vi "GyroDataStreamOut.vi"(11 "MockGyroData":T1={"BufferUpdateFIFO"="MockGyroBufferUpdate", "MockGyroCommandInput"="ModbusSubnetEGyroRxDataFIFO", "MockGyroDataOutput"="ModbusSubnetEGyroTxDataFIFO", "MockGyroDataRate"="MockGyroDataRateRegister", "MockGyroXValue"="MockGyroXValueRegister", "MockGyroYValue"="MockGyroYValueRegister", "MockGyroZValue"="MockGyroZValueRegister", "MockGyroStatus"="MockGyroStatusRegister", "MockGyroTemperature"="MockGyroTemperatureRegister", "CRCDataFIFO"="MockGyroCRCDataFIFO", "CRCCalculateFIFO"="MockGyroCRCCalculateFIFO", "CRCFIFO"="MockGyroCRCFIFO", "MockGyroCommandReplyFIFO"="MockGyroCommandReplyFIFO", "MockGyroReplyReadyFIFO"="MockGyroReplyReadyFIFO", "MockGyroModeFIFO"="MockGyroModeFIFO"}) -> ()   [LabVIEW 2016, in "FPGAMockGyro.lvlib"]
uses:
  FPGAMockGyro.lvlib
  DataTypes/MockGyroData.ctl
  DataTypes/MockGyroState.ctl
  DataTypes/MockGyroStateTypes.ctl
  DataTypes/MockGyroModes.ctl
  <vilib>/Platform/TimedLoop/XDataNode/timing_clust.ctl
  <vilib>/Platform/TimedLoop/XDataNode/nitl_modes.ctl
  <vilib>/Platform/TimedLoop/XDataNode/wakeup.ctl
  <vilib>/rvi/Emulation/niFpgaSctlEmulationGetInTimedLoop.vi
  <vilib>/rvi/Emulation/niFpgaEmulationReportErrorSimple.vi
  <vilib>/rvi/Emulation/niFpgaGetClockAttributes.vi
  <vilib>/rvi/Emulation/niFpgaCriticalErrorInLSC.vi
  <vilib>/rvi/DataTransferAndStorage/Container/Common/niFpgaContainerExecOnDevCompGetState.vi
  <vilib>/rvi/Emulation/niFpgaEmulationIsFPGAContextNoSignature.vi
  <vilib>/rvi/errors/niFpgaSetErrorForExecOnDevCompSimple.vi
  <vilib>/rvi/eio/common/nirviEmuReportErrorAndStop.vi
  <vilib>/rvi/DataTransferAndStorage/Container/Common/niFpgaContainerGetUniqueNameForEmu.vi
  <vilib>/rvi/FIFO/Fifo_Resource/nirvififoEmulationSetSize.vi
  <vilib>/rvi/FIFO/Fifo_Resource/nirviFifoEmulationQueueMgr.vi
  <instcachedir>/0/nirviFifoEmulationQueueMgr_E5CAEC123FF24DC58D834DCA3CDAA9B5.lvgen/nirviFifoEmulationQueueMgr_E5CAEC123FF24DC58D834DCA3CDAA9B5_000.vi
  <vilib>/rvi/FIFO/Fifo_Resource/nirvififoEmulationDetermineInputValidOut.vi
  <vilib>/rvi/FIFO/Fifo_Resource/nirvififoEmulationCreateLock.vi
  <vilib>/rvi/Emulation/niFpgaProcessEmulError.vi
  <vilib>/rvi/FIFO/Fifo_Resource/nirvififoEmulationObtainLock.vi
  <vilib>/rvi/FIFO/Fifo_Resource/nirvififoEmulationReleaseLock.vi
  <vilib>/rvi/occurrence/nirviWaitOnOccurrenceBase.vi
  <vilib>/rvi/errors/nirviReportUnexpectedCaseInternalError.vi
  <vilib>/rvi/errors/nirviReportUnexpectedCaseInternalError (U32).vi
  <vilib>/Utility/error.llb/Clear Errors.vi
  <vilib>/rvi/interface/RandomDataEmulation/niFpgaRandomDataHandleErrors.vi
  <vilib>/rvi/Memory/Memory_Emulation/niFpgaMemoryEmulationCacheClearOnFirstRun.vi
  <vilib>/rvi/Memory/Memory_Emulation/nirvimemoryEmulationManagerCache_MakeExclusive.vi
  <vilib>/rvi/Memory/Memory_Emulation/niFpgaMemoryEmulationValidateCache.vi
  <vilib>/rvi/Memory/Memory_Emulation/nirvimemoryEmulationManagerCache_InsertValue.vi
  <vilib>/rvi/Memory/Memory_Emulation/nirvimemoryEmulationManagerCache_ReleaseExclusive.vi
  <vilib>/rvi/Memory/Memory_Emulation/nirvimemoryEmulationManagerCache_GetValue.vi
  <vilib>/rvi/Memory/Memory_Emulation/nirvimemoryEmulationManagerCache_SetValue.vi
  <instcachedir>/0/nirviFifoEmulationQueueMgr_E5CAEC123FF24DC58D834DCA3CDAA9B5.lvgen/nirviFifoEmulationQueueMgr_E5CAEC123FF24DC58D834DCA3CDAA9B5_002.vi
  <instcachedir>/0/nirviFifoEmulationQueueMgr_E5CAEC123FF24DC58D834DCA3CDAA9B5.lvgen/nirviFifoEmulationQueueMgr_E5CAEC123FF24DC58D834DCA3CDAA9B5_001.vi
  <vilib>/Platform/TimedLoop/XDataNode/XDataNode.xnode
  <vilib>/rvi/DataTransferAndStorage/Container/XNode/niFpgaContainer.xnode
  <vilib>/rvi/FIFO/Fifo_Resource/niFpgaFifoEmulationRefIn.vi
  <vilib>/rvi/DataTransferAndStorage/Register/Emulation/niFpgaRegisterEmulationRefIn.vi
  <vilib>/Platform/TimedLoop/XDataNode/XDNodeRunTimeDep.lvlib
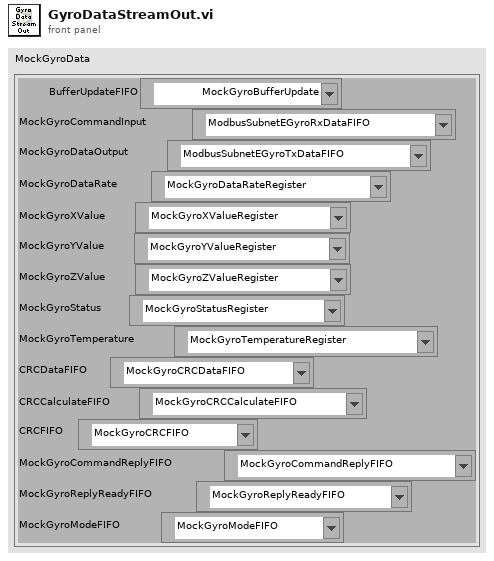
[diagram p1: front panel]
types:
  T1 = typedef "FPGAMockGyro.lvlib/MockGyroData.ctl" = cluster{"BufferUpdateFIFO":refnum<k21>, "MockGyroCommandInput":refnum<k21>, "MockGyroDataOutput":refnum<k21>, "MockGyroDataRate":refnum<k21>, "MockGyroXValue":refnum<k21>, "MockGyroYValue":refnum<k21>, "MockGyroZValue":refnum<k21>, "MockGyroStatus":refnum<k21>, "MockGyroTemperature":refnum<k21>, "CRCDataFIFO":refnum<k21>, "CRCCalculateFIFO":refnum<k21>, "CRCFIFO":refnum<k21>, "MockGyroCommandReplyFIFO":refnum<k21>, "MockGyroReplyReadyFIFO":refnum<k21>, "MockGyroModeFIFO":refnum<k21>}
  T2 = typedef "FPGAMockGyro.lvlib/MockGyroState.ctl" = cluster{"MockGyroStateTypes":T3, "DelayTicks":u64, "NextDelayTicks":u64, "Index":i32, "DataOutputArray":u8[], "MockGyroModes":T4}
  T3 = typedef "FPGAMockGyro.lvlib/MockGyroStateTypes.ctl" = enum8{"Processing", "WriteXValues", "WriteYValues", "WriteZValues", "WriteTemperature", "WriteDataOutput", "WriteCRC32", "Delaying", "CheckCommandReply", "WriteCommandReply", "Config"}
  T4 = typedef "FPGAMockGyro.lvlib/MockGyroModes.ctl" = enum8{"Normal", "Config"}
  T5 = typedef "XDNodeRunTimeDep.lvlib/timing_clust.ctl" = cluster{"Expected End [f-1]":u64, "Actual End [f-1]":u64, "Finished Late? [f-1]":bool, "Expected End [i-1]":u64, "Actual End [i-1]":u64, "Finished Late? [i-1]":bool, "Expected Start [i]":u64, "Actual Start [i]":u64, "Expected Start [f]":u64, "Actual Start [f]":u64, "Source Name":string, "Structure Name":string, "Period":i64, "Deadline":i64, "Offset":i64, "Start":i64, "Priority":i32, "Timeout":i32, "Mode":T6, "Wakeup Reason":T7, "Error":errorcluster, "Source Type":string, "Secondary Source Type":string, "Global End Time":u64, "Global Start Time":u64, "Frame Duration":u64, "Iteration Duration":u64, "Assigned CPU":i32, "I/O Scan Engine Mode":u32}
  T6 = typedef "XDNodeRunTimeDep.lvlib/nitl_modes.ctl" = enum32{"No Change", "Process missed periods, maintain original phase", "Discard missed periods, maintain original phase", "Process missed periods, ignore original phase", "Discard missed periods, ignore original phase"}
  T7 = typedef "XDNodeRunTimeDep.lvlib/wakeup.ctl" = enum32{"Normal", "Aborted", "Asynchronous wakeup", "Timing source error", "Timed loop error", "Timeout"}
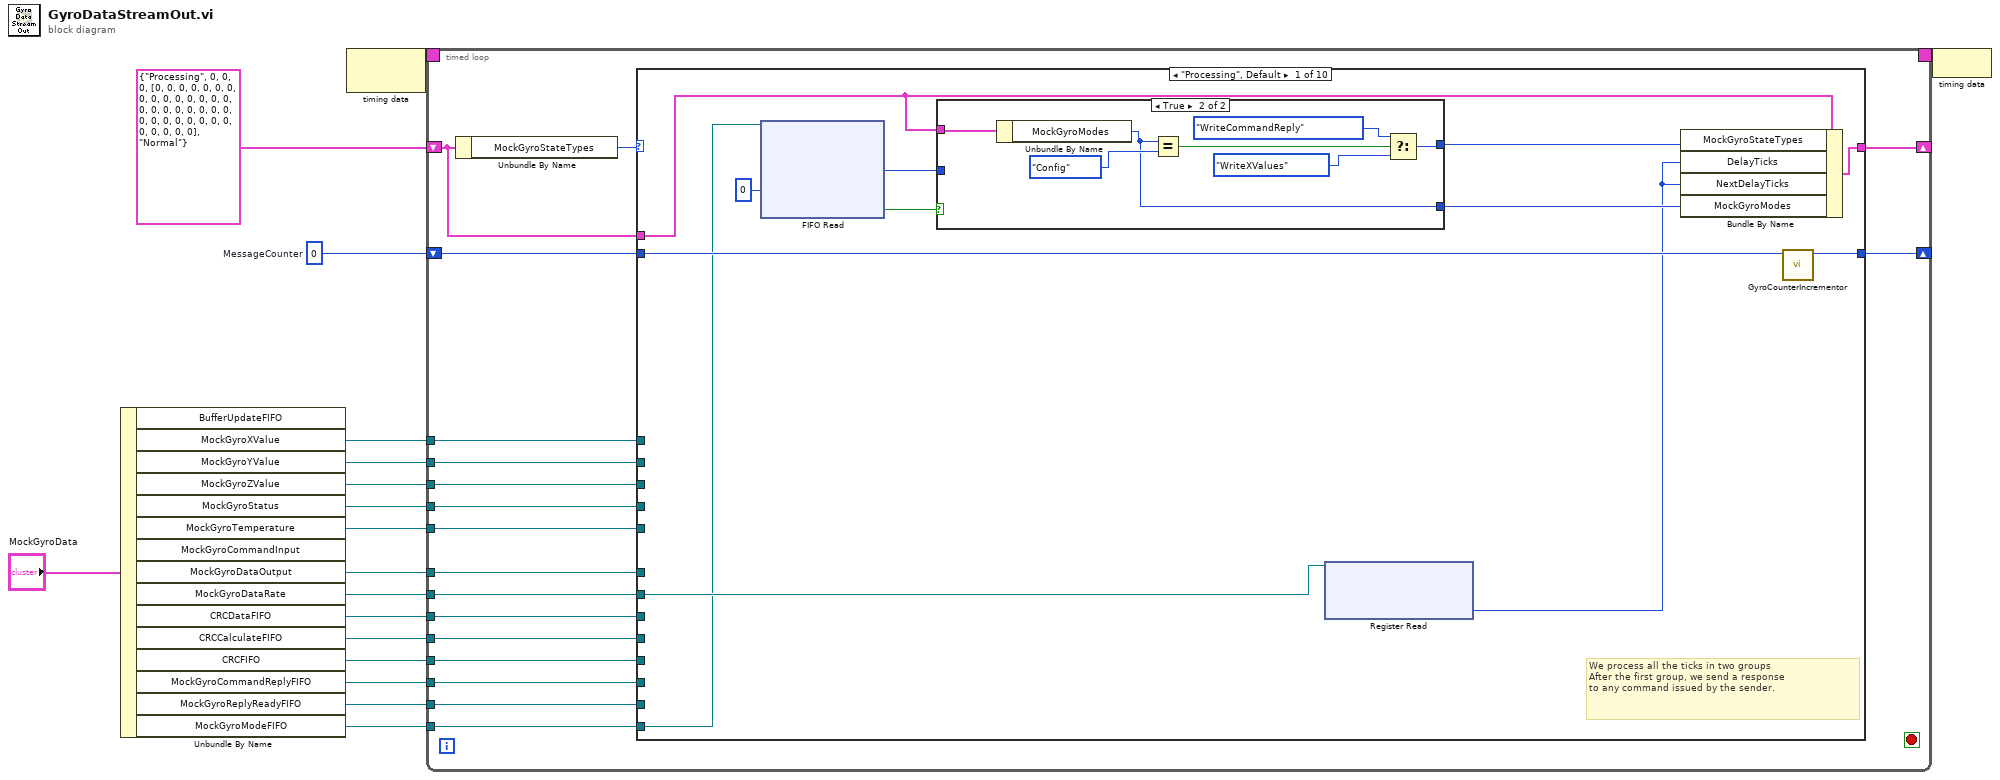
[diagram p0: block diagram]
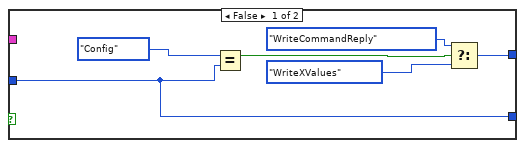
[diagram p2: hidden frame]
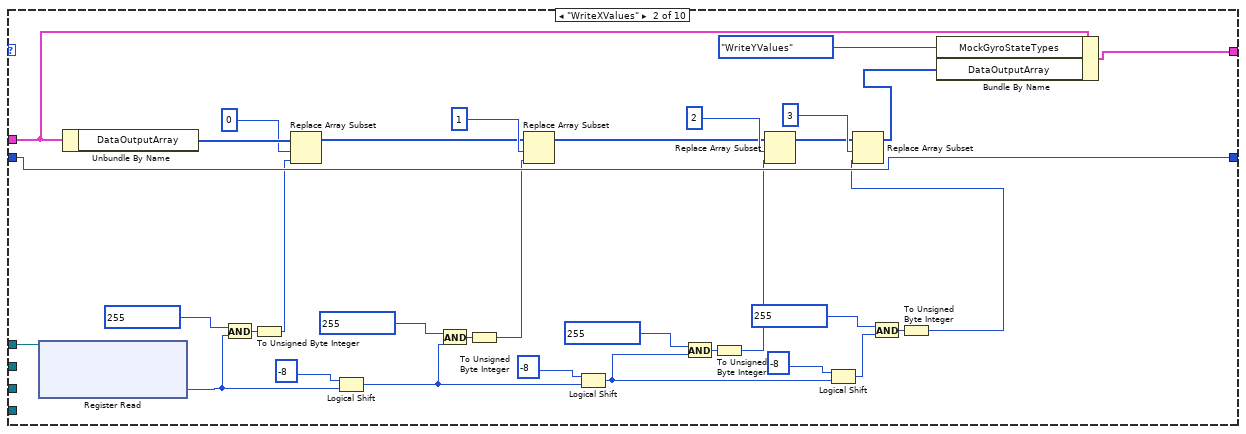
[diagram p3: hidden frame]
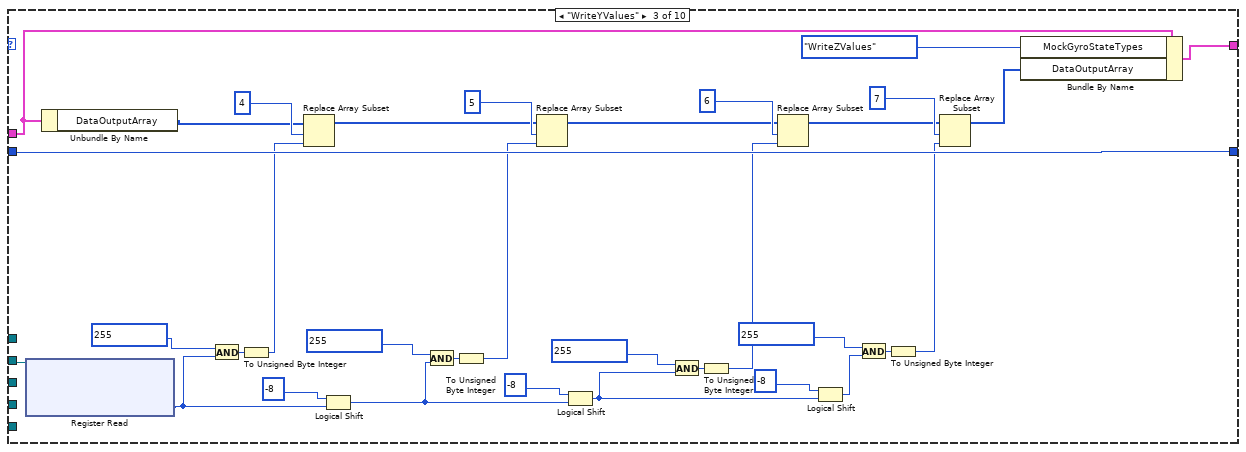
[diagram p4: hidden frame]
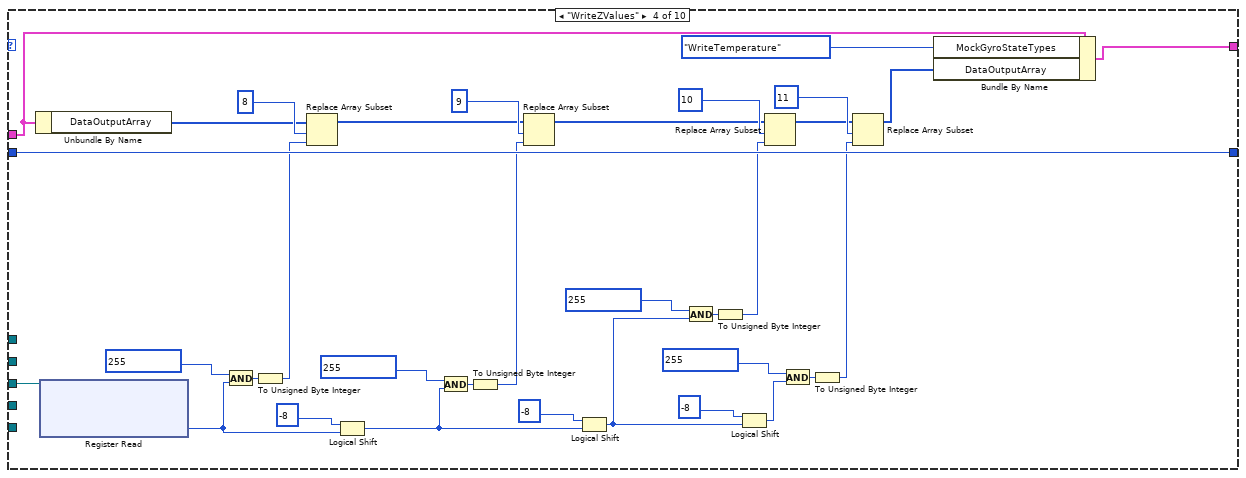
[diagram p5: hidden frame]
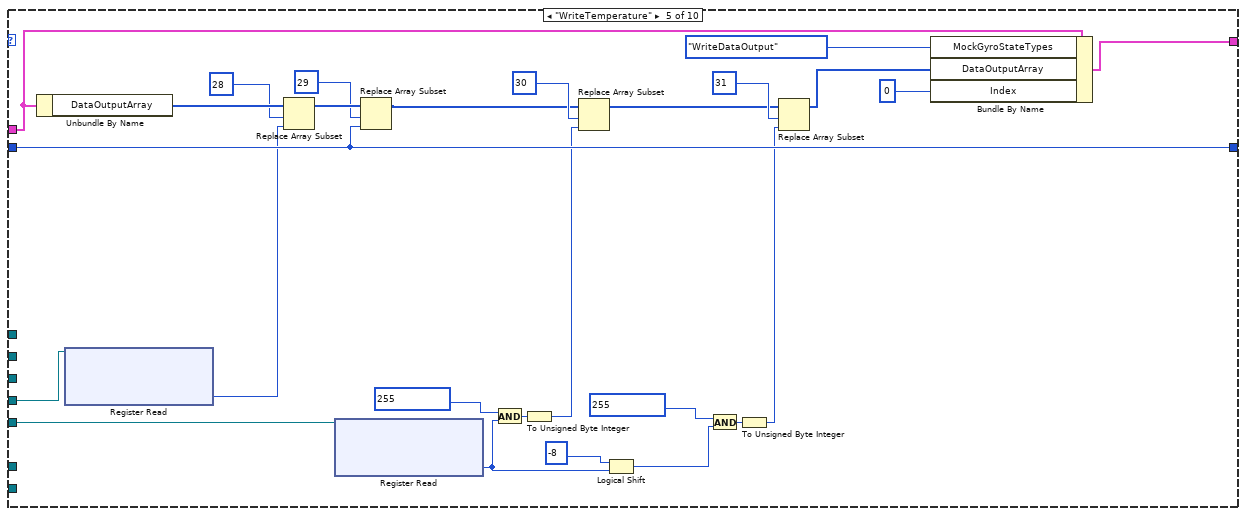
[diagram p6: hidden frame]
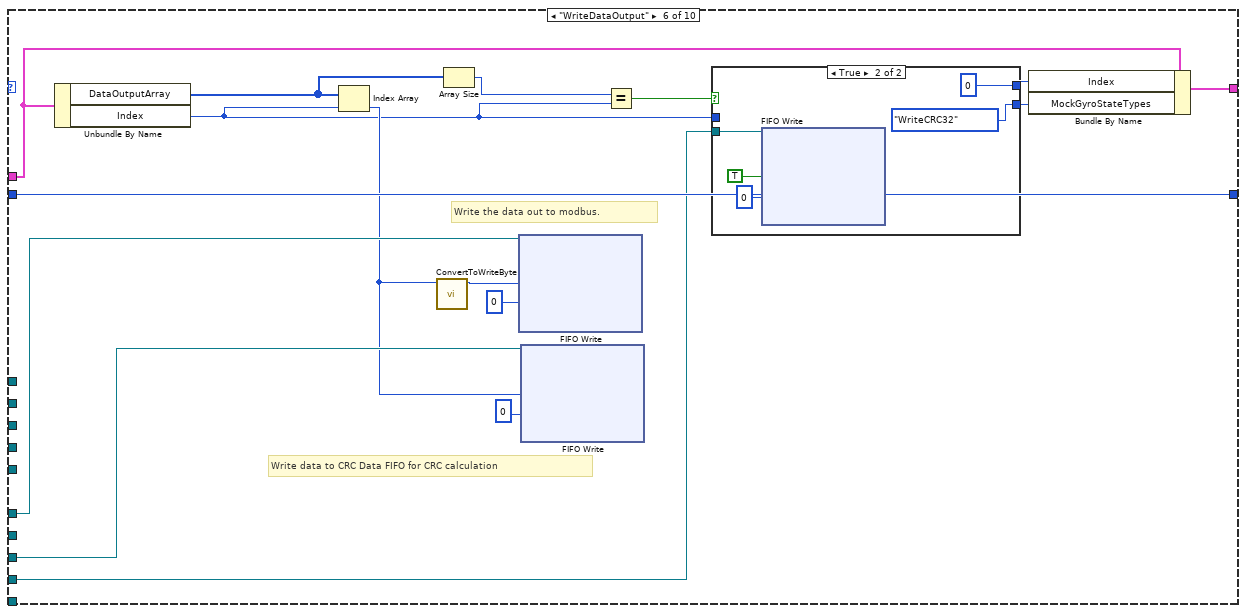
[diagram p7: hidden frame]
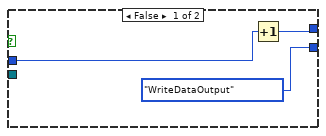
[diagram p8: hidden frame]
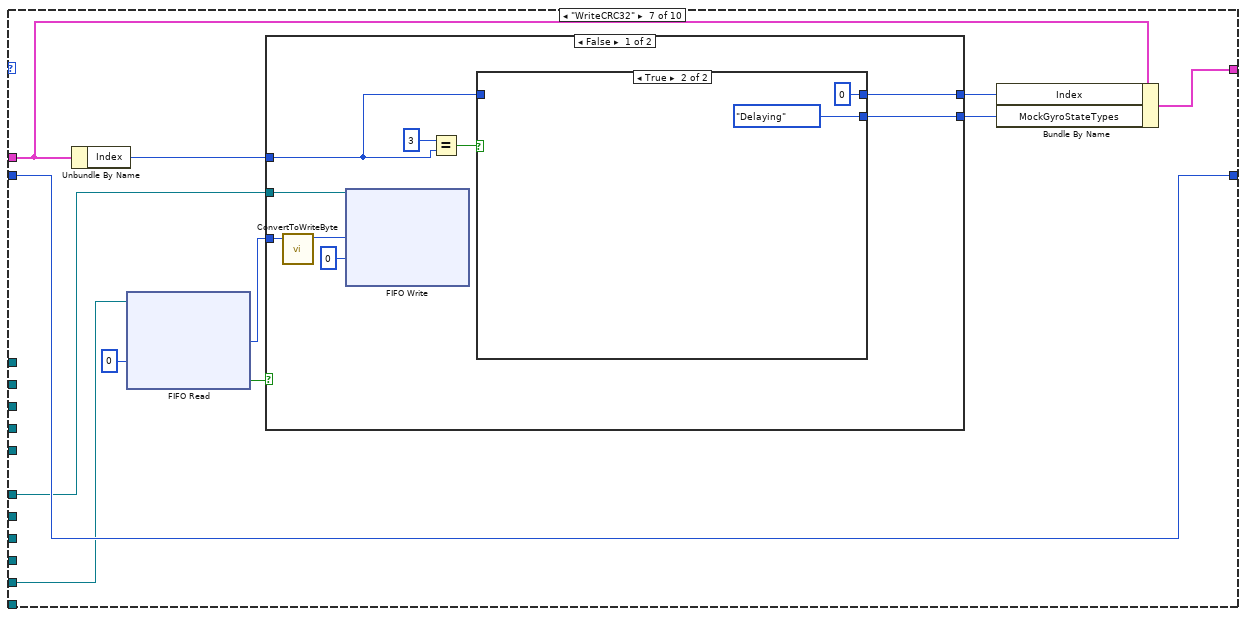
[diagram p9: hidden frame]
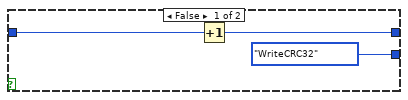
[diagram p10: hidden frame]
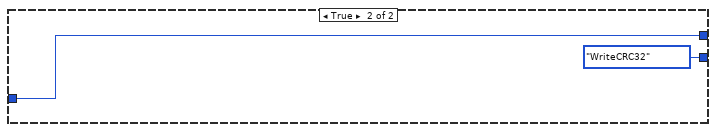
[diagram p11: hidden frame]
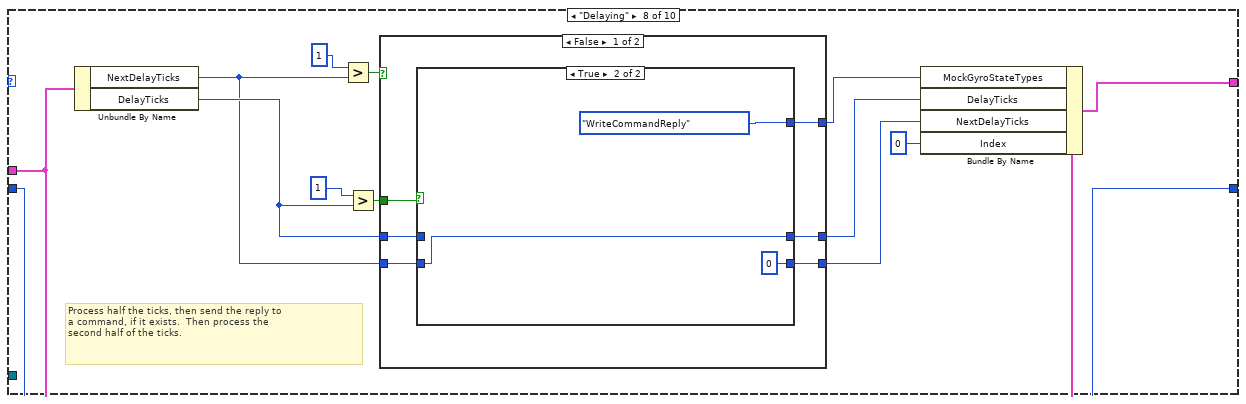
[diagram p12: hidden frame]
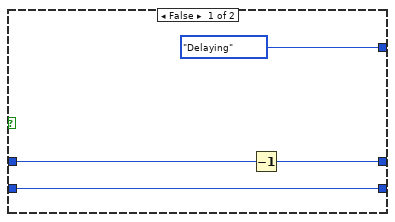
[diagram p13: hidden frame]
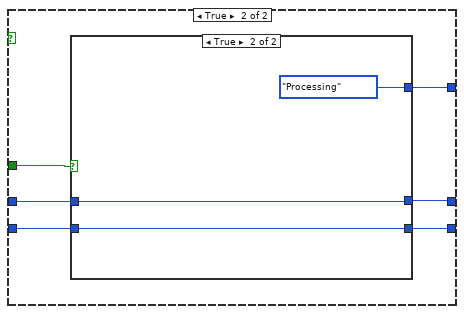
[diagram p14: hidden frame]
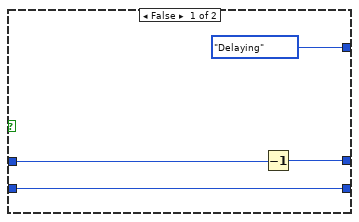
[diagram p15: hidden frame]
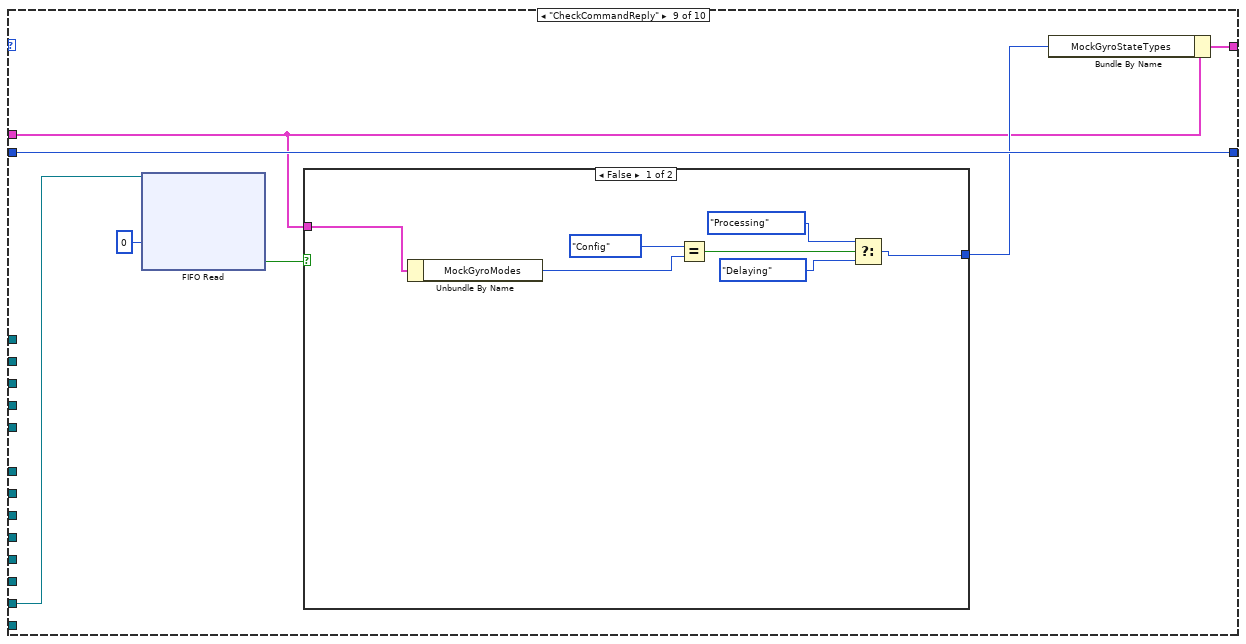
[diagram p16: hidden frame]
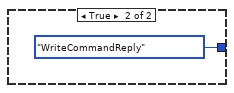
[diagram p17: hidden frame]
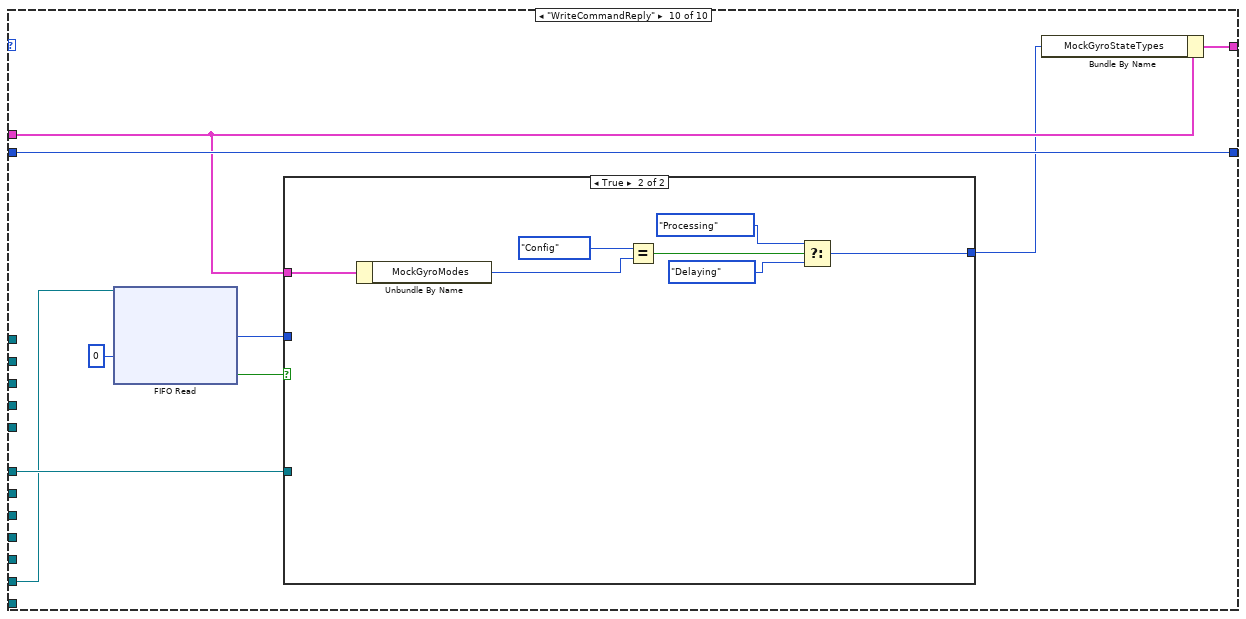
[diagram p18: hidden frame]
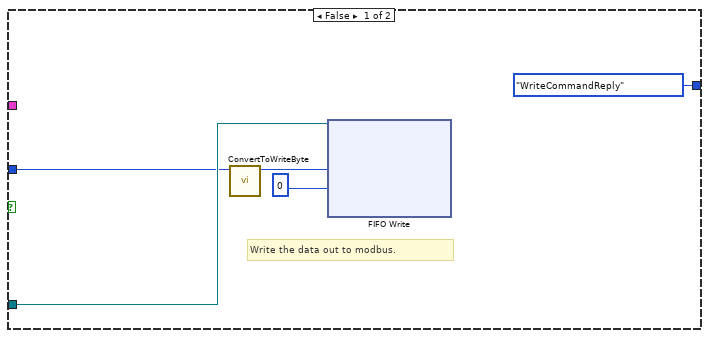
[diagram p19: hidden frame]
diagram:
  w18 = u8 0  # MessageCounter
  n1 = Unbundle By Name("MockGyroData") -> ("MockGyroXValue"=w11:refnum<k21>, "MockGyroYValue"=w10:refnum<k21>, "MockGyroZValue"=w9:refnum<k21>, "MockGyroStatus"=w8:refnum<k21>, "MockGyroTemperature"=w7:refnum<k21>, "MockGyroDataOutput"=w13:refnum<k21>, "MockGyroDataRate"=w14:refnum<k21>, "CRCDataFIFO"=w6:refnum<k21>, "CRCCalculateFIFO"=w5:refnum<k21>, "CRCFIFO"=w4:refnum<k21>, "MockGyroCommandReplyFIFO"=w3:refnum<k21>, "MockGyroReplyReadyFIFO"=w2:refnum<k21>, "MockGyroModeFIFO"=w1:refnum<k21>)  [unwired: 2 out]
  n2 = node-c288() -> (w16:T5)  [unwired: 1 in]
  n3 = timed-loop {
    shift-right: [w32] -> _
    shift-left: T2 {"MockGyroStateTypes"=enum."Processing", "DelayTicks"=0, "NextDelayTicks"=0, "Index"=0, "DataOutputArray"=[0, 0, 0, 0, 0, 0, 0, 0, 0, 0, 0, 0, 0, 0, 0, 0, 0, 0, 0, 0, 0, 0, 0, 0, 0, 0, 0, 0, 0, 0, 0, 0, 0, 0, 0, 0], "MockGyroModes"=enum."Normal"} ("MockGyroState") -> [w33]
    shift-right: [w36] -> _
    shift-left: w18 -> [w35]
    timing: w16 -> [_]
    timing-out: [_] -> w15
    tunnel: w14 -> [w31]
    tunnel: w13 -> [w30]
    tunnel: w11 -> [w29]
    tunnel: w10 -> [w28]
    tunnel: w9 -> [w27]
    tunnel: w8 -> [w26]
    tunnel: w7 -> [w25]
    tunnel: w6 -> [w24]
    tunnel: w5 -> [w23]
    tunnel: w4 -> [w22]
    tunnel: w3 -> [w21]
    tunnel: w2 -> [w20]
    tunnel: w1 -> [w19]
    stop <- _ stop-if-true
    n4 = Unbundle By Name(w33) -> ("MockGyroStateTypes"=w34:T3)
    n5 = case shown="\"Processing\", Default" w34 {
      tunnel: [w48 w83 w120 w153 w181 w196 w220 w250 w280 w298] -> w36
      tunnel: w35 -> [w47 w83 w120 w153 w181 w196 w220 w250 w280 w298]
      tunnel: w33 -> [w39 w86 w118 w151 w186 w195 w221 w249 w277 w293]
      tunnel: [w46 w85 w116 w149 w185 w197 w211 w248 w279 w299] -> w32
      tunnel: w31 -> [w44 _ _ _ _ _ _ _ _ _]
      tunnel: w30 -> [_ _ _ _ _ w200 w213 _ _ w300]
      tunnel: w29 -> [_ w81 _ _ _ _ _ _ _ _]
      tunnel: w28 -> [_ _ w99 _ _ _ _ _ _ _]
      tunnel: w27 -> [_ _ _ w132 _ _ _ _ _ _]
      tunnel: w26 -> [_ _ _ _ w163 _ _ _ _ _]
      tunnel: w25 -> [_ _ _ _ w166 _ _ _ _ _]
      tunnel: w24 -> [_ _ _ _ _ w194 _ _ _ _]
      tunnel: w23 -> [_ _ _ _ _ w187 _ _ _ _]
      tunnel: w22 -> [_ _ _ _ _ _ w216 _ _ _]
      tunnel: w21 -> [_ _ _ _ _ _ _ _ _ w297]
      tunnel: w20 -> [_ _ _ _ _ _ _ _ w283 _]
      tunnel: w19 -> [w43 _ _ _ _ _ _ _ _ _]
      frame "Processing", Default {
        # "We process all the ticks in two groups\nAfter the first group, we send a response\nto any command issued by the sender."
        n6 = xnode ("FIFO Read")("Timeout"=0, "FIFO In"=w43) -> ("Element"=w40:u8, "Timed Out?"=w41:bool)  [unwired: 1 out]
        n7 = case shown="True" w41 {
          tunnel: [w51 w55] -> w45
          tunnel: w40 -> [w49 _]
          tunnel: w39 -> [_ w60]
          tunnel: [w49 w56] -> w38
          frame False {
            n8 = Equal?(x=MockGyroModes."Config" ("MockGyroModes"), y=w49) -> (x = y?=w54:bool)
            n9 = Select(t=MockGyroStateTypes."WriteCommandReply" ("MockGyroStateTypes"), s=w54, f=MockGyroStateTypes."WriteXValues") -> (s? t:f=w51:T3)
          }
          frame True {
            n10 = Unbundle By Name(w60) -> ("MockGyroModes"=w56:T4)
            n11 = Equal?(x=w56, y=MockGyroModes."Config" ("MockGyroModes")) -> (x = y?=w61:bool)
            n12 = Select(t=MockGyroStateTypes."WriteCommandReply" ("f"), s=w61, f=MockGyroStateTypes."WriteXValues") -> (s? t:f=w55:T3)
          }
        }
        n13 = xnode ("Register Read")("Register In"=w44) -> ("Data"=w37:u64)  [unwired: 1 out]
        n14 = Bundle By Name(cluster=w39, "MockGyroStateTypes"=w45, "DelayTicks"=w37, "NextDelayTicks"=w37, "MockGyroModes"=w38) -> (w46:T2)
        n15 = call "GyroCounterIncrementor.vi"("CurrentCounter"=w47) -> ("NewCounter"=w48:u8)  [unwired: 10 in]
      }
      frame "WriteXValues" {
        n16 = xnode ("Register Read")("Register In"=w81) -> ("Data"=w78:u32)  [unwired: 1 out]
        n17 = Unbundle By Name(w86) -> ("DataOutputArray"=w94:u8[])
        n18 = And(x=u32 255, y=w78) -> (x .and. y?=w79:u32)
        n19 = To Unsigned Byte Integer(number=w79) -> (unsigned 8bit integer=w76:u8)
        n20 = Replace Array Subset(array=w94, new element=w76, index=0) -> (w89:u8[])
        n21 = Logical Shift(y=i16 -8, x=w78) -> (x << y=w71:u32)
        n22 = And(x=u32 255, y=w71) -> (x .and. y?=w74:u32)
        n23 = To Unsigned Byte Integer(number=w74) -> (unsigned 8bit integer=w73:u8)
        n24 = Replace Array Subset(array=w89, new element=w73, index=1) -> (w88:u8[])
        n25 = Logical Shift(y=i16 -8, x=w71) -> (x << y=w64:u32)
        n26 = And(x=u32 255, y=w64) -> (x .and. y?=w70:u32)
        n27 = To Unsigned Byte Integer(number=w70) -> (unsigned 8bit integer=w65:u8)
        n28 = Replace Array Subset(array=w88, new element=w65, index=2) -> (w87:u8[])
        n29 = Logical Shift(y=i16 -8, x=w64) -> (x << y=w63:u32)
        n30 = And(x=u32 255, y=w63) -> (x .and. y?=w67:u32)
        n31 = To Unsigned Byte Integer(number=w67) -> (unsigned 8bit integer=w62:u8)
        n32 = Replace Array Subset(array=w87, new element=w62, index=3) -> (w84:u8[])
        n33 = Bundle By Name(cluster=w86, "MockGyroStateTypes"=MockGyroStateTypes."WriteYValues", "DataOutputArray"=w84) -> (w85:T2)
      }
      frame "WriteYValues" {
        n34 = xnode ("Register Read")("Register In"=w99) -> ("Data"=w112:u32)  [unwired: 1 out]
        n35 = Unbundle By Name(w118) -> ("DataOutputArray"=w119:u8[])
        n36 = And(x=u32 255, y=w112) -> (x .and. y?=w113:u32)
        n37 = To Unsigned Byte Integer(number=w113) -> (unsigned 8bit integer=w98:u8)
        n38 = Replace Array Subset(array=w119, new element=w98, index=4) -> (w123:u8[])
        n39 = Logical Shift(y=i16 -8, x=w112) -> (x << y=w107:u32)
        n40 = And(x=u32 255, y=w107) -> (x .and. y?=w109:u32)
        n41 = To Unsigned Byte Integer(number=w109) -> (unsigned 8bit integer=w97:u8)
        n42 = Replace Array Subset(array=w123, new element=w97, index=5) -> (w122:u8[])
        n43 = Logical Shift(y=i16 -8, x=w107) -> (x << y=w101:u32)
        n44 = And(x=u32 255, y=w101) -> (x .and. y?=w106:u32)
        n45 = To Unsigned Byte Integer(number=w106) -> (unsigned 8bit integer=w96:u8)
        n46 = Replace Array Subset(array=w122, new element=w96, index=6) -> (w121:u8[])
        n47 = Logical Shift(y=i16 -8, x=w101) -> (x << y=w100:u32)
        n48 = And(x=u32 255, y=w100) -> (x .and. y?=w103:u32)
        n49 = To Unsigned Byte Integer(number=w103) -> (unsigned 8bit integer=w95:u8)
        n50 = Replace Array Subset(array=w121, new element=w95, index=7) -> (w117:u8[])
        n51 = Bundle By Name(cluster=w118, "MockGyroStateTypes"=MockGyroStateTypes."WriteZValues", "DataOutputArray"=w117) -> (w116:T2)
      }
      frame "WriteZValues" {
        n52 = Unbundle By Name(w151) -> ("DataOutputArray"=w152:u8[])
        n53 = xnode ("Register Read")("Register In"=w132) -> ("Data"=w145:u32)  [unwired: 1 out]
        n54 = And(x=u32 255, y=w145) -> (x .and. y?=w146:u32)
        n55 = To Unsigned Byte Integer(number=w146) -> (unsigned 8bit integer=w131:u8)
        n56 = Replace Array Subset(array=w152, new element=w131, index=8) -> (w156:u8[])
        n57 = Logical Shift(y=i16 -8, x=w145) -> (x << y=w140:u32)
        n58 = And(x=u32 255, y=w140) -> (x .and. y?=w142:u32)
        n59 = To Unsigned Byte Integer(number=w142) -> (unsigned 8bit integer=w130:u8)
        n60 = Replace Array Subset(array=w156, new element=w130, index=9) -> (w155:u8[])
        n61 = Logical Shift(y=i16 -8, x=w140) -> (x << y=w134:u32)
        n62 = And(x=u32 255, y=w134) -> (x .and. y?=w139:u32)
        n63 = To Unsigned Byte Integer(number=w139) -> (unsigned 8bit integer=w129:u8)
        n64 = Logical Shift(y=i16 -8, x=w134) -> (x << y=w133:u32)
        n65 = Replace Array Subset(array=w155, new element=w129, index=10) -> (w154:u8[])
        n66 = And(x=u32 255, y=w133) -> (x .and. y?=w136:u32)
        n67 = To Unsigned Byte Integer(number=w136) -> (unsigned 8bit integer=w128:u8)
        n68 = Replace Array Subset(array=w154, new element=w128, index=11) -> (w150:u8[])
        n69 = Bundle By Name(cluster=w151, "MockGyroStateTypes"=MockGyroStateTypes."WriteTemperature", "DataOutputArray"=w150) -> (w149:T2)
      }
      frame "WriteTemperature" {
        n70 = Unbundle By Name(w186) -> ("DataOutputArray"=w183:u8[])
        n71 = xnode ("Register Read")("Register In"=w163) -> ("Data"=w162:u8)  [unwired: 1 out]
        n72 = Replace Array Subset(array=w183, new element=w162, index=28) -> (w180:u8[])
        n73 = xnode ("Register Read")("Register In"=w166) -> ("Data"=w171:u16)  [unwired: 1 out]
        n74 = Replace Array Subset(array=w180, new element=w181, index=29) -> (w176:u8[])
        n75 = And(x=u16 255, y=w171) -> (x .and. y?=w172:u16)
        n76 = To Unsigned Byte Integer(number=w172) -> (unsigned 8bit integer=w164:u8)
        n77 = Replace Array Subset(array=w176, new element=w164, index=30) -> (w175:u8[])
        n78 = Logical Shift(y=i16 -8, x=w171) -> (x << y=w167:u16)
        n79 = And(x=u16 255, y=w167) -> (x .and. y?=w168:u16)
        n80 = To Unsigned Byte Integer(number=w168) -> (unsigned 8bit integer=w165:u8)
        n81 = Replace Array Subset(array=w175, new element=w165, index=31) -> (w174:u8[])
        n82 = Bundle By Name(cluster=w186, "MockGyroStateTypes"=MockGyroStateTypes."WriteDataOutput", "DataOutputArray"=w174, "Index"=u8 0) -> (w185:T2)
      }
      frame "WriteDataOutput" {
        # "Write data to CRC Data FIFO for CRC calculation"
        # "Write the data out to modbus."
        n83 = Unbundle By Name(w195) -> ("DataOutputArray"=w198:u8[], "Index"=w188:i32)
        n84 = Index Array(array=w198, index=w188) -> (element=w192:u8)
        n85 = call "ConvertToWriteByte.vi"("Input"=w192) -> ("Output"=w199:u16)  [unwired: 10 in]
        n86 = Array Size(array=w198) -> (size(s)=w202:i32)
        n87 = xnode ("FIFO Write")("Element"=w199, "Timeout"=0, "FIFO In"=w200) -> ()  [unwired: 2 out]
        n88 = xnode ("FIFO Write")("Element"=w192, "Timeout"=0, "FIFO In"=w194) -> ()  [unwired: 2 out]
        n89 = Equal?(x=w202, y=w188) -> (x = y?=w189:bool)
        n90 = case shown="True" w189 {
          tunnel: [w203 0] -> w191
          tunnel: [MockGyroStateTypes."WriteDataOutput" ("MockGyroStateTypes") MockGyroStateTypes."WriteCRC32" ("MockGyroStateTypes")] -> w190
          tunnel: w188 -> [w204 _]
          tunnel: w187 -> [_ w208]
          frame False {
            n91 = Increment(x=w204) -> (x+1=w203:i32)
          }
          frame True {
            n92 = xnode ("FIFO Write")("Element"=TRUE, "Timeout"=0, "FIFO In"=w208) -> ()  [unwired: 2 out]
          }
        }
        n93 = Bundle By Name(cluster=w195, "Index"=w191, "MockGyroStateTypes"=w190) -> (w197:T2)
      }
      frame "WriteCRC32" {
        n94 = Unbundle By Name(w221) -> ("Index"=w219:i32)
        n95 = xnode ("FIFO Read")("Timeout"=0, "FIFO In"=w216) -> ("Element"=w212:u8, "Timed Out?"=w214:bool)  [unwired: 1 out]
        n96 = case shown="False" w214 {
          tunnel: w219 -> [w228 w237]
          tunnel: [w227 w237] -> w218
          tunnel: [w226 MockGyroStateTypes."WriteCRC32" ("MockGyroStateTypes")] -> w217
          tunnel: w213 -> [w225 _]
          tunnel: w212 -> [w223 _]
          frame False {
            n97 = call "ConvertToWriteByte.vi"("Input"=w223) -> ("Output"=w222:u16)  [unwired: 10 in]
            n98 = xnode ("FIFO Write")("Element"=w222, "Timeout"=0, "FIFO In"=w225) -> ()  [unwired: 2 out]
            n99 = Equal?(x=3, y=w228) -> (x = y?=w230:bool)
            n100 = case shown="True" w230 {
              tunnel: w228 -> [w233 _]
              tunnel: [w232 0] -> w227
              tunnel: [MockGyroStateTypes."WriteCRC32" ("MockGyroStateTypes") MockGyroStateTypes."Delaying" ("MockGyroStateTypes")] -> w226
              frame False {
                n101 = Increment(x=w233) -> (x+1=w232:i32)
              }
              frame True {
              }
            }
          }
          frame True {
          }
        }
        n102 = Bundle By Name(cluster=w221, "Index"=w218, "MockGyroStateTypes"=w217) -> (w211:T2)
      }
      frame "Delaying" {
        # "Process half the ticks, then send the reply to \na command, if it exists.  Then process the \nsecond half of the ticks."
        n103 = Unbundle By Name(w249) -> ("NextDelayTicks"=w243:u64, "DelayTicks"=w245:u64)
        n104 = Greater?(x=u64 1, y=w243) -> (0:w240:bool)
        n105 = Greater?(x=u64 1, y=w245) -> (0:w239:bool)
        n106 = case shown="False" w240 {
          tunnel: w245 -> [w256 w266]
          tunnel: [w255 w265] -> w244
          tunnel: w243 -> [w254 w267]
          tunnel: [w253 w268] -> w242
          tunnel: w239 -> [w252 w269]
          tunnel: [w251 w264] -> w238
          frame False {
            n107 = case shown="True" w252 {
              tunnel: w256 -> [w260 _]
              tunnel: [w259 w262] -> w255
              tunnel: w254 -> [w258 w262]
              tunnel: [w258 u64 0 ("NextDelayTicks")] -> w253
              tunnel: [MockGyroStateTypes."Delaying" ("f") MockGyroStateTypes."WriteCommandReply" ("MockGyroStateTypes")] -> w251
              frame False {
                n108 = Decrement(x=w260) -> (x-1=w259:u64)
              }
              frame True {
              }
            }
          }
          frame True {
            n109 = case shown="True" w269 {
              tunnel: [w273 w276] -> w268
              tunnel: w267 -> [w273 w276]
              tunnel: w266 -> [w272 w274]
              tunnel: [w271 w274] -> w265
              tunnel: [MockGyroStateTypes."Delaying" ("f") MockGyroStateTypes."Processing" ("f")] -> w264
              frame False {
                n110 = Decrement(x=w272) -> (x-1=w271:u64)
              }
              frame True {
              }
            }
          }
        }
        n111 = Bundle By Name(cluster=w249, "MockGyroStateTypes"=w238, "DelayTicks"=w244, "NextDelayTicks"=w242, "Index"=0) -> (w248:T2)
      }
      frame "CheckCommandReply" {
        n112 = xnode ("FIFO Read")("Timeout"=0, "FIFO In"=w283) -> ("Timed Out?"=w281:bool)  [unwired: 2 out]
        n113 = case shown="False" w281 {
          tunnel: [w284 MockGyroStateTypes."WriteCommandReply" ("MockGyroStateTypes")] -> w278
          tunnel: w277 -> [w285 _]
          frame False {
            n114 = Unbundle By Name(w285) -> ("MockGyroModes"=w286:T4)
            n115 = Equal?(x=MockGyroModes."Config", y=w286) -> (x = y?=w288:bool)
            n116 = Select(t=MockGyroStateTypes."Processing", s=w288, f=MockGyroStateTypes."Delaying" ("MockGyroStateTypes")) -> (s? t:f=w284:T3)
          }
          frame True {
          }
        }
        n117 = Bundle By Name(cluster=w277, "MockGyroStateTypes"=w278) -> (w279:T2)
      }
      frame "WriteCommandReply" {
        n118 = xnode ("FIFO Read")("Timeout"=0, "FIFO In"=w297) -> ("Element"=w294:u8, "Timed Out?"=w295:bool)  [unwired: 1 out]
        n119 = case shown="True" w295 {
          tunnel: w300 -> [w305 _]
          tunnel: w294 -> [w302 _]
          tunnel: w293 -> [_ w307]
          tunnel: [MockGyroStateTypes."WriteCommandReply" ("MockGyroStateTypes") w306] -> w292
          frame False {
            # "Write the data out to modbus."
            n120 = call "ConvertToWriteByte.vi"("Input"=w302) -> ("Output"=w303:u16)  [unwired: 10 in]
            n121 = xnode ("FIFO Write")("Element"=w303, "Timeout"=0, "FIFO In"=w305) -> ()  [unwired: 2 out]
          }
          frame True {
            n122 = Unbundle By Name(w307) -> ("MockGyroModes"=w308:T4)
            n123 = Equal?(x=MockGyroModes."Config", y=w308) -> (x = y?=w310:bool)
            n124 = Select(t=MockGyroStateTypes."Processing", s=w310, f=MockGyroStateTypes."Delaying" ("MockGyroStateTypes")) -> (s? t:f=w306:T3)
          }
        }
        n125 = Bundle By Name(cluster=w293, "MockGyroStateTypes"=w292) -> (w299:T2)
      }
    }
  }
  n126 = node-c288(w15) -> ()
